vi "mainUI.vi"() -> ()   [LabVIEW 2024]
panel:
  out "error out":errorcluster
  in  "Stop Button 2":bool
  in  "Stop Button":bool
  in  "Play":bool
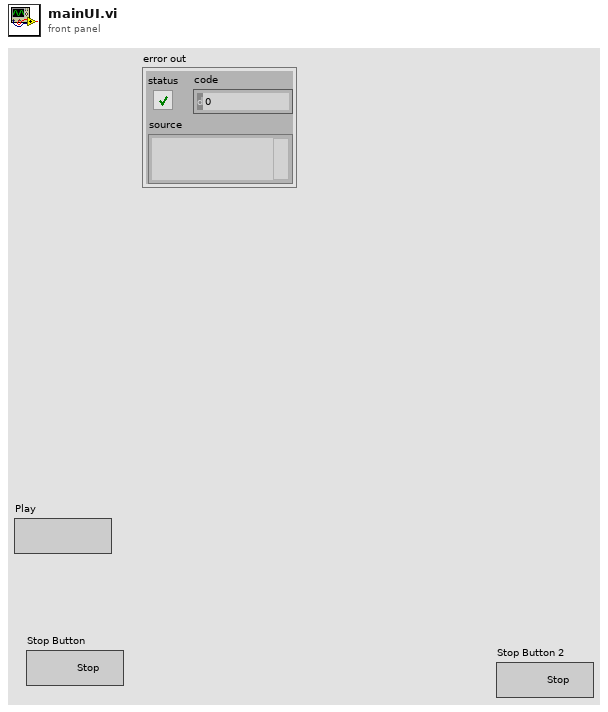
[diagram p1: front panel]
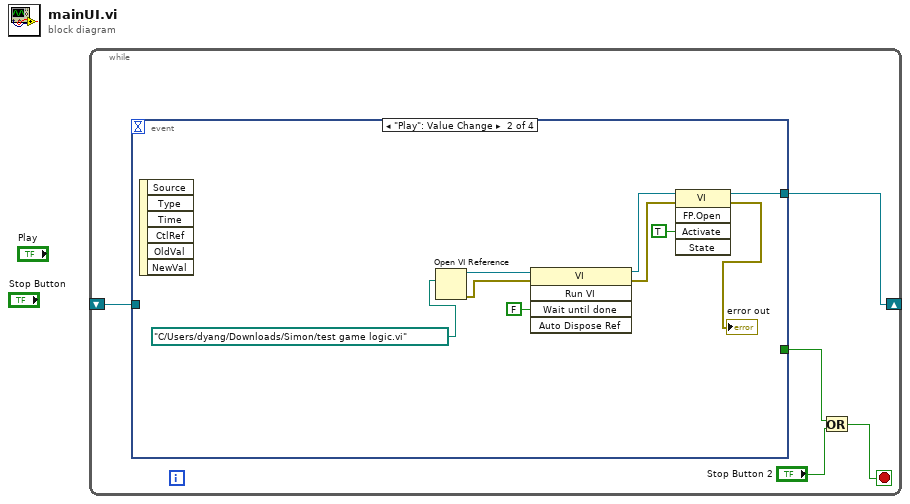
[diagram p0: block diagram]
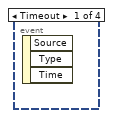
[diagram p2: hidden frame]
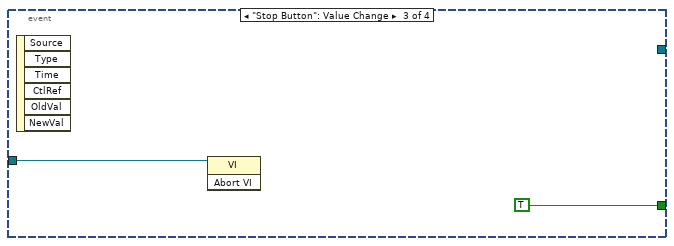
[diagram p3: hidden frame]
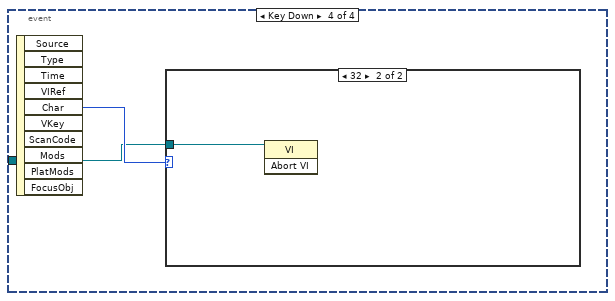
[diagram p4: hidden frame]
diagram:
  n1 = while {
    shift-right: [w4] -> _
    shift-left: _ -> [w5]
    stop <- w3 stop-if-true
    n2 = event shown="[1] \"Play\": Value Change" {
      selector: _ -> [_ _ _ _]
      dyn-events: _ -> [_ _ _ _]
      timeout: _ -> [_ _ _ _]
      tunnel: w5 -> [_ _ w16 w17]
      tunnel: [_ w9 _ _] -> w4
      tunnel: [_ _ TRUE _] -> w1
      event Timeout {
        n3 = event-data() -> ()  [unwired: 1 in, 3 out]
      }
      event "Play": Value Change {
        n4 = event-data() -> ()  [unwired: 1 in, 6 out]
        n5 = Open VI Reference(vi path=path "C:/Users/dyang/Downloads/Simon/test game logic.vi") -> (vi reference=w14:refnum<vi>, error out=w11:errorcluster)  [unwired: 5 in]
        n6 = invoke class="VI" method="Run VI"(reference=w14, error in=w11, "Wait until done"=FALSE ("Wait Until Done")) -> (reference out=w10:refnum<vi>, error out=w8:errorcluster)  [unwired: 2 in, 3 out]
        n7 = invoke class="VI" method="FP.Open"(reference=w10, error in=w8, "Activate"=TRUE ("Activate?")) -> (reference out=w9:refnum<vi>, error out=→"error out":errorcluster)  [unwired: 2 in, 3 out]
      }
      event "Stop Button": Value Change {
        n8 = event-data() -> ()  [unwired: 1 in, 6 out]
        n9 = invoke class="VI" method="Abort VI"(reference=w16) -> ()  [unwired: 2 in, 3 out]
      }
      event Key Down {
        n10 = event-data() -> ("Char"=w18:i16)  [unwired: 1 in, 9 out]
        n11 = case shown="32" w18 {
          tunnel: w17 -> [_ w19]
          frame 0, Default {
          }
          frame 32 {
            n12 = invoke class="VI" method="Abort VI"(reference=w19) -> ()  [unwired: 2 in, 3 out]
          }
        }
      }
    }
    n13 = Or(x=w1, y="Stop Button 2") -> (x .or. y?=w3:bool)
  }
